vi "Draw BG Image.vi"(6 "Control Ref Queue":T4, 8 "error in (no error)":errorcluster, 10 "Multiplot Representation In":T1, 11 "2D Error Bar.lvclass in":refnum<class "2D Error Bar.lvclass">) -> (0 "error out":errorcluster, 2 "Multiplot Representation Out":T1, 3 "2D Error Bar.lvclass out":refnum<class "2D Error Bar.lvclass">)   [LabVIEW 2020, in "2D Error Bar.lvclass"]
uses:
  <vilib>/Math Plots/2D Math Plots/2D Error Bar/2D Error Bar/2D Error Bar.lvclass
  <vilib>/Math Plots/2D Math Plots/2D Plot/Action String/2DMathPlot Ctrl Act Queue.ctl
  <vilib>/Math Plots/2D Math Plots/2D Plot/Action String/2DMathPlot Ctrl Act Cluster.ctl
  <vilib>/Math Plots/2D Math Plots/2D Plot/Action String/2DMathPlot State Class.ctl
  e:/builds/penguin/labview/branches/2020/dev/dist/vi.lib/Math Plots/2D Math Plots/2D Plot/2D Plot/2D Plot.lvclass
  <vilib>/Math Plots/2D Math Plots/2D Plot/2D Plot/Typedef/Multiplot Representation.ctl
  <vilib>/Math Plots/2D Math Plots/2D Plot/2D Plot/Typedef/Plot Representation.ctl
  <vilib>/Math Plots/2D Math Plots/2D Plot/2D Plot/Typedef/Range Cluster.ctl
  <vilib>/Math Plots/2D Math Plots/2D Error Bar/2D Error Bar/2D Error Bar.lvclass/2D Error Bar.ctl
  <vilib>/Math Plots/2D Math Plots/2D Plot/2D Plot/2D Plot.lvclass
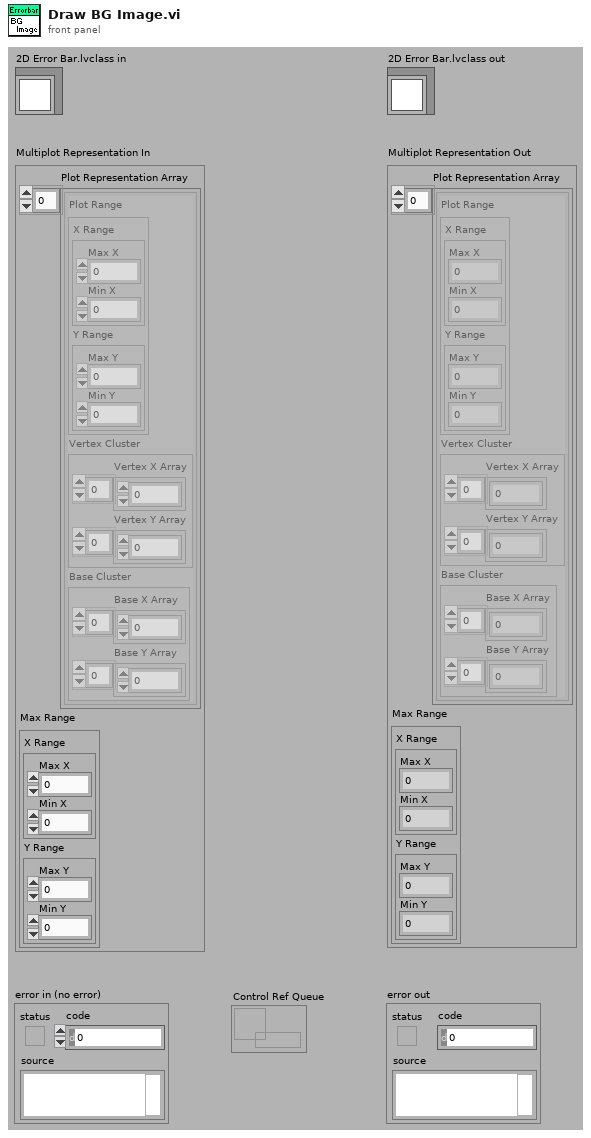
[diagram p1: front panel]
types:
  T1 = typedef "2D Plot.lvclass/Multiplot Representation.ctl" = cluster{"Plot Representation Array":T2[], "Max Range":T3}
  T2 = typedef "2D Plot.lvclass/Plot Representation.ctl" = cluster{"Plot Range":T3, "Vertex Cluster":cluster{"Vertex X Array":dbl[], "Vertex Y Array":dbl[]}, "Base Cluster":cluster{"Base X Array":dbl[], "Base Y Array":dbl[]}}
  T3 = typedef "2D Plot.lvclass/Range Cluster.ctl" = cluster{"X Range":cluster{"Max X":dbl, "Min X":dbl}, "Y Range":cluster{"Max Y":dbl, "Min Y":dbl}}
  T4 = typedef "2DMathPlot Ctrl Act Queue.ctl" = refnum<queue>
  T5 = typedef "2D Error Bar.lvclass/2D Error Bar Property Array.ctl" = T6[]
  T6 = typedef "2D Error Bar.lvclass/2D Error Bar Property.ctl" = cluster{"Marker Size":dbl, "Marker Line Style":u8, "Marker Line Width":u8, "Marker Color":u32, "Error Bar Interpolation":enum16{"Show Point", "Show Line", "Show Bar"}, "Error Mode":enum16{"Show Y Error", "Show X Error", "Show Both Error"}}
  T7 = typedef "2DMathPlot Ctrl Act Cluster.ctl" = cluster{"Plot Area Ref":refnum<vi>, "Z Axis Ref":refnum<vi>, "Legend Ref":refnum<vi>, "XControl Ref":refnum<vi>, "Facade Ref":refnum<vi>, "Display State Change Class":T8}
  T8 = typedef "2DMathPlot State Class.ctl" = enum16{"Update All (Undo)", "Update General", "Update Appearance", "Update Format", "Update Scale", "Update Marker", "Update Cursor", "None"}
  T9 = enum16{"Show Y Error", "Show X Error", "Show Both Error"}
  T10 = cluster{"Width":u16, "Style":enum32{"Solid", "Dash", "Dot", "DashDot", "DashDotDot"}}
  T11 = cluster{"Base X Array":dbl[], "Base Y Array":dbl[]}
  T12 = cluster{"Vertex X Array":dbl[], "Vertex Y Array":dbl[]}
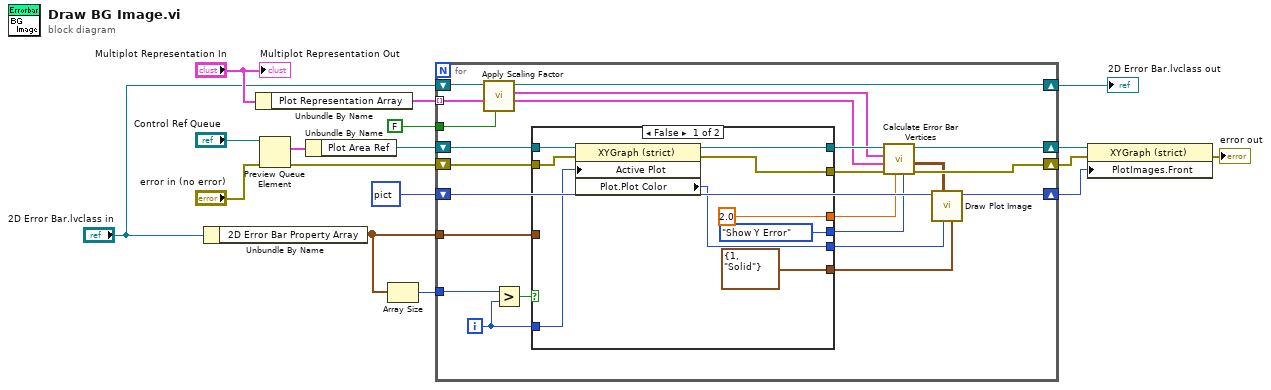
[diagram p0: block diagram]
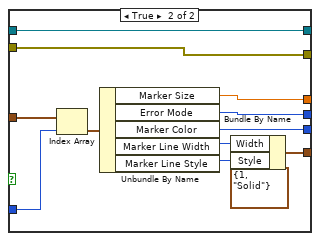
[diagram p2: hidden frame]
diagram:
  n1 = Unbundle By Name("2D Error Bar.lvclass in") -> ("2D Error Bar Property Array"=w1:T5)
  n2 = Unbundle By Name("Multiplot Representation In") -> ("Plot Representation Array"=w13:T2[])
  n3 = Preview Queue Element(queue="Control Ref Queue", error in (no error)="error in (no error)") -> (element=w17:T7, error out=w7:errorcluster)  [unwired: 3 out]
  n4 = Unbundle By Name(w17) -> ("Plot Area Ref"=w9:refnum<vi>)
  n5 = Array Size(array=w1) -> (size(s)=w5:i32)
  n6 = for {
    tunnel: w13 -> [w26] mode=indexing
    shift-right: [w18] -> w11
    shift-left: picture data[5B] ("Picture In") -> [w37]
    tunnel: w1 -> [w40]
    shift-right: [w39] -> w8
    shift-left: w9 -> [w32]
    shift-right: [w38] -> w6
    shift-left: w7 -> [w30]
    tunnel: w5 -> [w34]
    shift-right: [w24] -> w3
    shift-left: "2D Error Bar.lvclass in" -> [w25]
    tunnel: FALSE ("Plot Image?") -> [w21]
    i -> [w33]
    n7 = call <vilib>:"Apply Scaling Factor.vi"("Apply to Vertex?"=w21, "Plot Representation Cluster"=w26, "2D Plot.lvclass in"=w25) -> ("Base Cluster"=w23:T11, "Vertex Cluster"=w22:T12, "2D Plot.lvclass out"=w24:refnum<class "2D Error Bar.lvclass">)  [unwired: 1 in, 5 out]
    n8 = Greater?(x=w34, y=w33) -> (0:w35:bool)
    n9 = case shown="False" w35 {
      tunnel: w40 -> [_ w61]
      tunnel: [w47 w58] -> w28
      tunnel: [T10 {"Width"=1, "Style"=enum."Solid"} ("pen") w57] -> w27
      tunnel: w33 -> [w46 w55]
      tunnel: w32 -> [w48 w53]
      tunnel: [w45 w53] -> w31
      tunnel: w30 -> [w44 w54]
      tunnel: [w43 w54] -> w29
      tunnel: [T9."Show Y Error" ("Error Mode") w51] -> w20
      tunnel: [2.0 ("Marker Size") w50] -> w19
      frame False {
        n10 = property class="XYGraph (strict)"(reference=w48, error in=w44, "Active Plot"=w46) -> (reference out=w45:refnum<vi>, error out=w43:errorcluster, "Plot.Plot Color"=w47:u32)
      }
      frame True {
        n11 = Index Array(array=w61, index=w55) -> (element=w52:T6)
        n12 = Unbundle By Name(w52) -> ("Marker Size"=w50:dbl, "Error Mode"=w51:T9, "Marker Color"=w58:u32, "Marker Line Width"=w60:u8, "Marker Line Style"=w59:u8)
        n13 = Bundle By Name(cluster=T10 {"Width"=1, "Style"=enum."Solid"} ("pen"), "Width"=w60, "Style"=w59) -> (w57:T10)
      }
    }
    n14 = call <vilib>:"Calculate Error Bar Vertices.vi"("Error Mode"=w20, "Marker Size"=w19, "error in (no error)"=w29, "Base Cluster"=w23, "Vertex Cluster"=w22, "Plot Area Ref"=w31) -> ("error out"=w38:errorcluster, "Error Bar Vertex"=w36:cluster{"X":i16, "Y":i16}[][], "Dup Plot Area Ref"=w39:refnum<vi>)  [unwired: 3 out]
    n15 = call <vilib>:"Draw Plot Image.vi"("pen"=w27, "Plot Color"=w28, "Plot Vertex"=w36, "Picture In"=w37) -> ("Picture Out"=w18:picture)  [unwired: 7 out]
  }
  "2D Error Bar.lvclass out" <- w3
  n16 = property class="XYGraph (strict)"(reference=w8, error in=w6, "PlotImages.Front"=w11) -> (error out=→"error out":errorcluster)  [unwired: 1 out]
  "Multiplot Representation Out" <- "Multiplot Representation In"
